vi "_DataPluginInitInfo.vi"(8 "error in (no error)":errorcluster) -> (0 "error out":errorcluster, 1 "Result Items":string[][](array[string]), 2 "Offline":bool, 3 "DataPlugin information out":T1[](array[typedef]), 10 "String":string="Loading DataPlugins from ni.com/dataplugins")   [LabVIEW 2020]
uses:
  <vilib>/Platform/storage/utility/DataPluginSynchronization/_DataPluginInfo.ctl
  <vilib>/Platform/storage/utility/DataPluginSynchronization/_localizeDataPluginMessageEnum.ctl
panel:
  out "Boolean":bool
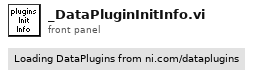
[diagram p1: front panel]
types:
  T1 = typedef "_DataPluginInfo.ctl" = cluster{"name":string, "status":u32, "extensions":string[], "description":string, "url":string, "lastExportTime":i64, "type":string, "version":string, "exist":bool, "current version":string, "model":string}
  T2 = typedef "_localizeDataPluginMessageEnum.ctl" = enum16{"Installed", "Not Installed", "Updates Available", "Latest version:", "Double click the \"Description\" cell.", "Install/Update DataPlugins", "Offline: ", "Please ensure that your network connection is working.", "No DataPlugins can be updated.", "Loading DataPlugins from ni.com/dataplugins", "Acquiring and installing ", "Install", "Update", "Succeed", "Failed", " Installation successful.", "Include *. to search for a file extension", "Current version:", " Installation failed.", "Installing update", "Update successful.", "Update failed.", "Updated", "Failed to update DataPlugins."}
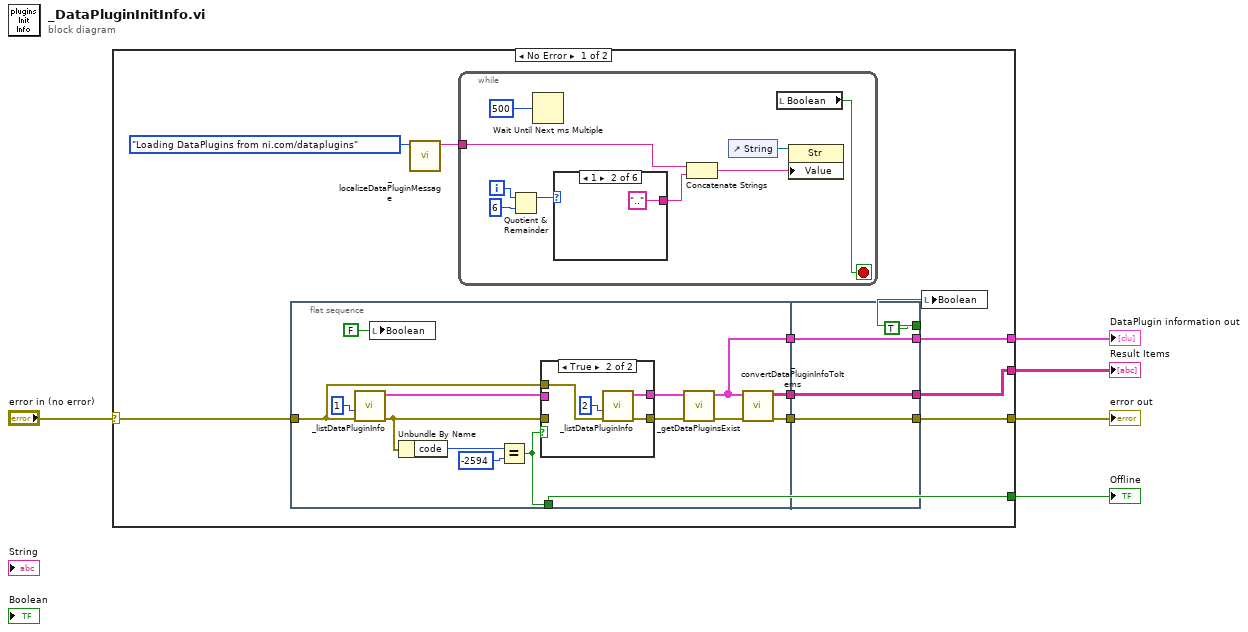
[diagram p0: block diagram]
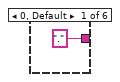
[diagram p2: hidden frame]
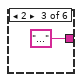
[diagram p3: hidden frame]
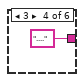
[diagram p4: hidden frame]
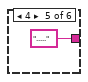
[diagram p5: hidden frame]
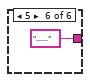
[diagram p6: hidden frame]
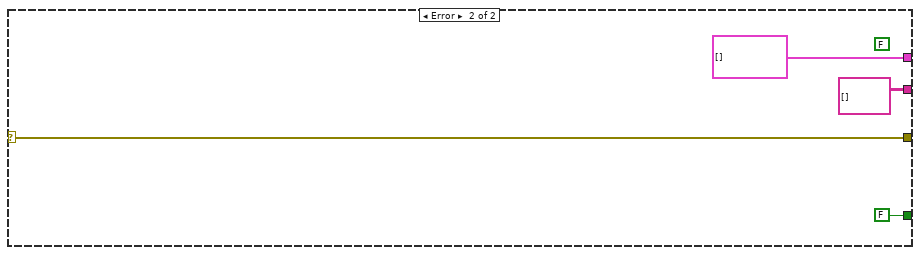
[diagram p8: hidden frame]
diagram:
  n1 = case shown="No Error" "error in (no error)" {
    selector: "error in (no error)" -> [w9 w57]
    tunnel: [w13 w57] -> w5
    tunnel: [w12 T1[] [] ("Web DataPlugin Info")] -> w4
    tunnel: [w11 string[][] [] ("Items")] -> w3
    tunnel: [w10 FALSE] -> w2
    frame No Error {
      n2 = flat-sequence {
        tunnel: w9 -> [w37]
        tunnel: [w34] -> w16
        tunnel: [w39] -> w15
        tunnel: [w41] -> w10
        tunnel: [w40] -> w14
        tunnel: [TRUE] -> w8
        tunnel: w16 -> [w53]
        tunnel: [w54] -> w13
        tunnel: w15 -> [w54]
        tunnel: [w53] -> w12
        tunnel: [w52] -> w11
        tunnel: w14 -> [w52]
        frame #0 {
          n3 = call <vilib>:"_listDataPluginInfo.vi"("error in (no error)"=w37, "source"=u32 1) -> ("error out"=w38:errorcluster, "DataPlugin information"=w42:T1[])  [unwired: 8 in]
          n4 = local write "Boolean"(FALSE ("Boolean")) -> ()
          n5 = Unbundle By Name(w38) -> ("code"=w44:i32)
          n6 = Equal?(x=w44, y=-2594) -> (x = y?=w41:bool)
          n7 = case shown="True" w41 {
            tunnel: [w47 w50] -> w35
            tunnel: [w46 w49] -> w33
            tunnel: w42 -> [w47 _]
            tunnel: w38 -> [w46 _]
            tunnel: w37 -> [_ w48]
            frame False {
            }
            frame True {
              n8 = call <vilib>:"_listDataPluginInfo.vi"("error in (no error)"=w48, "source"=u32 2) -> ("error out"=w49:errorcluster, "DataPlugin information"=w50:T1[])  [unwired: 8 in]
            }
          }
          n9 = call <vilib>:"_getDataPluginsExist.vi"("error in (no error)"=w33, "DataPlugin information in"=w35) -> ("error out"=w32:errorcluster, "DataPlugin information out"=w34:T1[])  [unwired: 8 in]
          n10 = call <vilib>:"_convertDataPluginInfoToItems.vi"("error in (no error)"=w32, "DataPlugin information"=w34) -> ("error out"=w39:errorcluster, "Items"=w40:string[][])  [unwired: 8 in]
        }
        frame #1 {
        }
      }
      n11 = call <vilib>:"_localizeDataPluginMessage.vi"("message in"=_localizeDataPluginMessageEnum."Loading DataPlugins from ni.com/dataplugins") -> ("message out"=w6:string)  [unwired: 10 in]
      n12 = while {
        tunnel: w6 -> [w18]
        i -> [w24]
        stop <- w25 stop-if-true
        n13 = Quotient & Remainder(x=w24, y=6) -> (x-y*floor(x/y)=w21:i32)  [unwired: 1 out]
        n14 = Wait Until Next ms Multiple(millisecond multiple=u32 500) -> ()  [unwired: 1 out]
        n15 = case shown="1" w21 {
          tunnel: ["." ("y") ".." ("y") "..." ("y") "...." ("y") "....." ("y") "......" ("y")] -> w22
          frame 0, Default {
          }
          frame 1 {
          }
          frame 2 {
          }
          frame 3 {
          }
          frame 4 {
          }
          frame 5 {
          }
        }
        n16 = Concatenate Strings(w18, w22) -> (w17:string)
        n17 = control-ref of="String"() -> (w19:refnum<vi>)
        n18 = local read "Boolean"() -> (w25:bool)
        n19 = property class="Str"(reference=w19, "Value"=w17) -> ()  [unwired: 1 in, 2 out]
      }
      n20 = local write "Boolean"(w8) -> ()
    }
    frame Error {
      (unwired) FALSE
    }
  }
  "error out" <- w5
  "Result Items" <- w3
  "DataPlugin information out" <- w4
  "Offline" <- w2
